vi "LLLL.vi"() -> ()   [LabVIEW 2016]
panel:
  in  "DEDO 5":dbl(knob) scale=0.0..100.0
  in  "DEDO 4":dbl(knob) scale=0.0..100.0
  in  "DEDO 3":dbl(knob) scale=0.0..100.0
  in  "DEDO 2":dbl(knob) scale=0.0..100.0
  in  "DEDO 1":dbl(knob) scale=0.0..100.0
  out "Waveform Chart":u32(graph)
  in  "Stop Button":bool
  out "Error Out":errorcluster
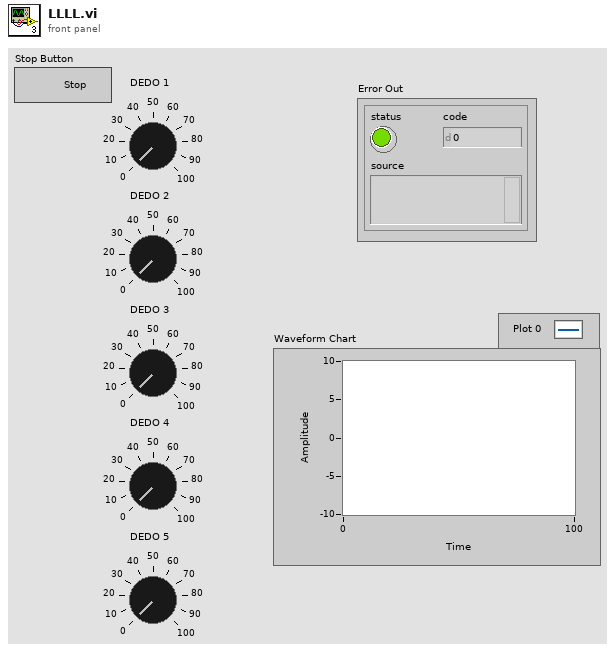
[diagram p1: front panel]
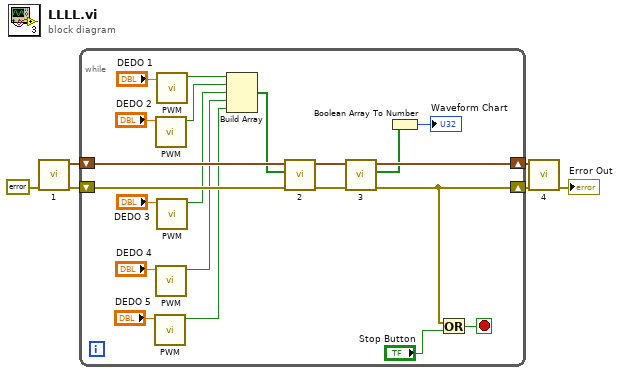
[diagram p0: block diagram]
diagram:
  n1 = call "1.vi"("Error In"=errorcluster {"status"=FALSE, "code"=0, "source"=""}) -> ("Error Out"=w6:errorcluster, "buffer"=w5:cluster{"PIPE in":i32, "PIPE OUT":i32})  [unwired: 9 in]
  n2 = while {
    shift-right: [w20] -> w3
    shift-left: w6 -> [w27]
    shift-right: [w24] -> w4
    shift-left: w5 -> [w26]
    stop <- w21 stop-if-true
    n3 = call "PWM.vi"("Knob"="DEDO 5") -> ("s? t:f"=w13:bool)  [unwired: 10 in]
    n4 = call "PWM.vi"("Knob"="DEDO 2") -> ("s? t:f"=w16:bool)  [unwired: 10 in]
    n5 = call "PWM.vi"("Knob"="DEDO 4") -> ("s? t:f"=w14:bool)  [unwired: 10 in]
    n6 = call "PWM.vi"("Knob"="DEDO 1") -> ("s? t:f"=w17:bool)  [unwired: 10 in]
    n7 = call "PWM.vi"("Knob"="DEDO 3") -> ("s? t:f"=w15:bool)  [unwired: 10 in]
    n8 = Build Array(w17, w16, w15, w14, w13) -> (w7:bool[])
    n9 = call <userlib>:"2.vi"("Error In"=w27, "Array"=w7, "buffer in"=w26) -> ("Error Out"=w23:errorcluster, "buffer out"=w25:cluster{"PIPE IN":i32, "PIPE OUT":i32})  [unwired: 7 in]
    n10 = call <userlib>:"3.vi"("Error In"=w23, "buffer in"=w25) -> ("Error Out"=w20:errorcluster, "lectura"=w18:bool[], "buffer out"=w24:cluster{"Pipe in":i32, "Pipe out":i32})  [unwired: 7 in]
    n11 = Boolean Array To Number(Boolean array=w18) -> (number=→"Waveform Chart":u32)
    n12 = Or(x=w20, y="Stop Button") -> (x .or. y?=w21:bool)
  }
  n13 = call <userlib>:"4.vi"("Error In"=w3, "buffer in"=w4) -> ("Error Out"=→"Error Out":errorcluster)  [unwired: 8 in, 1 out]
